vi "ReadType_Bar_AF.vi"(6 "error in":errorcluster, 11 "File Bar":string="C:\\Users\\Hung\\Desktop\\RawData\\New Raw") -> (0 "Linear Velocity (m/s)":dbl, 1 "Gain Max":dbl, 2 "Gain Min":dbl, 3 "Type":i16, 4 "error out":errorcluster, 5 "Linear Move Distance (m)":dbl)   [LabVIEW 2020]
panel:
  out "x/y":dbl
  out "D_Magnetic (mm)":dbl
  out "Simulated Distance":dbl
  out "Duration":dbl
  out "Waveform Graph":dbl[](graph)
  out "V_ship (m/s)":dbl
  out "Voltage Response":dbl
  out "Simulated Distance":i16
  out "D_Magnetic(mm)":i16
  out "Duration":u16
  out "Max ABS Magnetic Value":dbl
  in  "Gain":dbl=1.0 min=-20.0 max=20.0
  out "Data_Double":dbl[](array[numeric])
  out "Number Sample":u32
  out "Size Data":i32
  out "data":i16[](array[numeric])
  in  "file path (use dialog) 2":path=path "C:/Users/Hung/Downloads/filewritefromGUI.bar"
  # "Type 2 is Move Motion\nType 1 is Change Kepco"
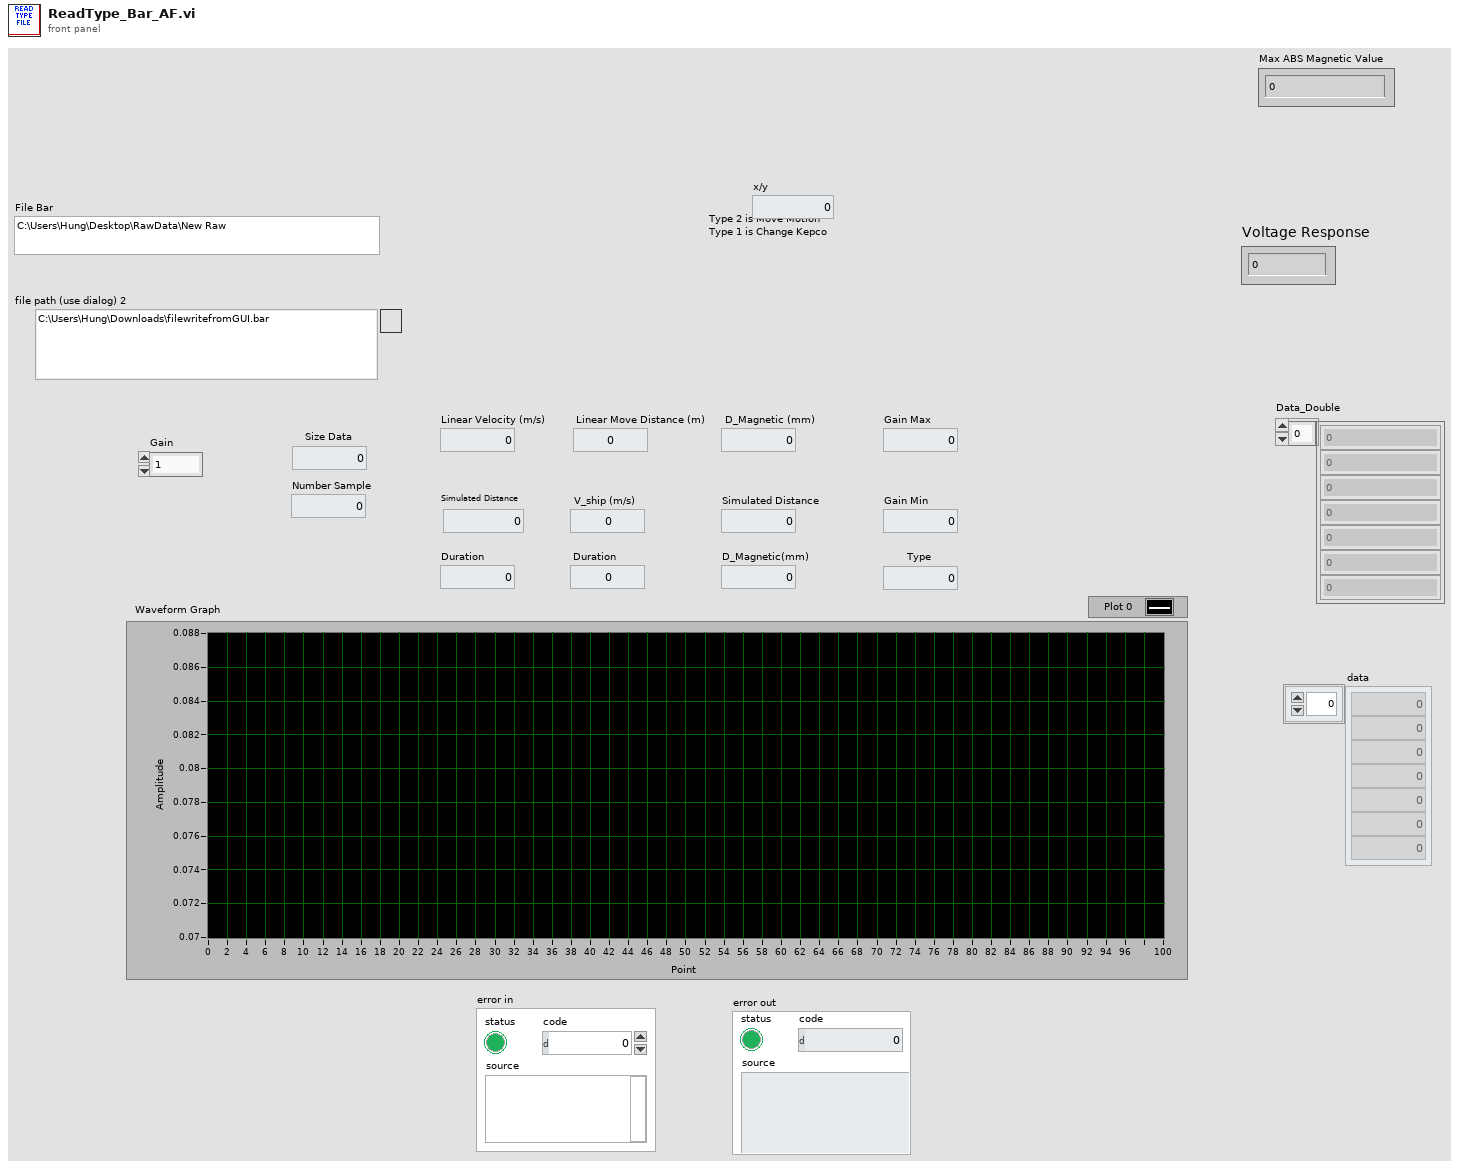
[diagram p1: front panel]
types:
  T1 = enum16{"big-endian, network order", "native, host order", "little-endian"}
  T2 = enum16{"open", "replace", "create", "open or create", "replace or create", "replace or create with confirmation"}
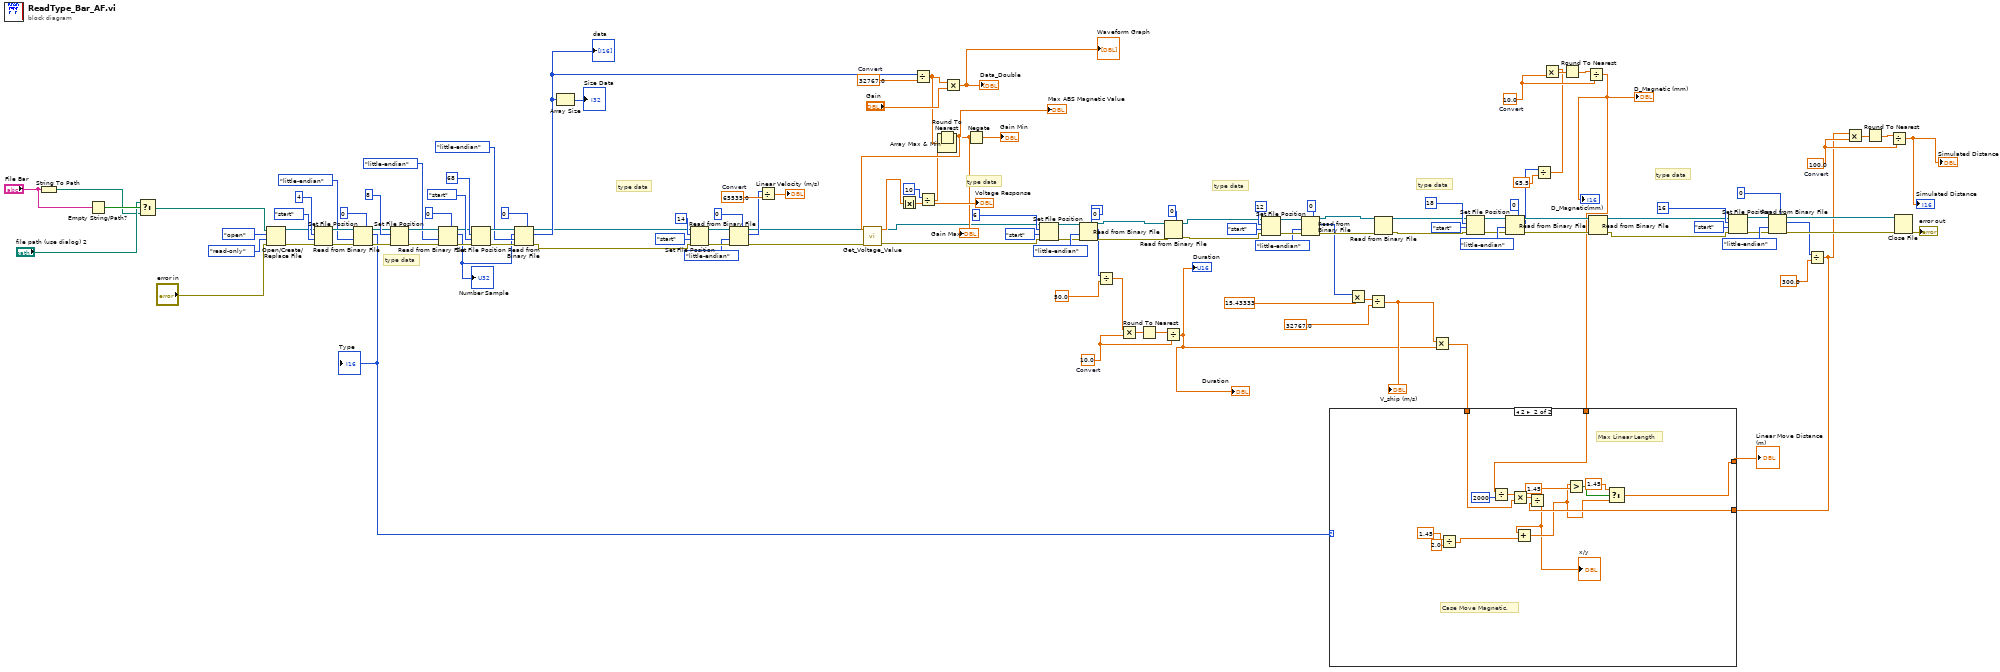
[diagram p0: block diagram]
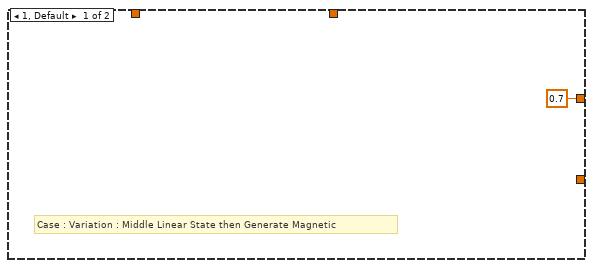
[diagram p2: hidden frame]
diagram:
  w10 = 10.0  # Convert
  w16 = 10.0  # Convert
  w17 = 100.0  # Convert
  w85 = 65535.0  # Convert
  w104 = 32767.0  # Convert
  # "type data"
  # "type data"
  # "type data"
  # "type data"
  # "type data"
  # "type data"
  n1 = String To Path(string="File Bar") -> (path=w26:path)
  n2 = Empty String/Path?(string/path="File Bar") -> (empty?=w28:bool)
  n3 = Select(t="file path (use dialog) 2", s=w28, f=w26) -> (s? t:f=w30:path)
  n4 = Open/Create/Replace File(file path (use dialog)=w30, error in="error in", operation (0:open)=T2."open", access (0:read/write)=enum16{"read/write", "read-only", "write-only"}."read-only") -> (refnum out=w62:refnum<file>, error out=w123:errorcluster)  [unwired: 2 in, 1 out]
  n5 = Set File Position(offset (in bytes) (0)=i64 4, refnum=w62, from (0:start)=enum16{"start", "end", "current"}."start", error in=w123) -> (refnum out=w124:refnum<file>, error out=w122:errorcluster)
  n6 = Read from Binary File(5:i16 0, 8:w122, 9:T1."little-endian" ("byte order (0:big-endian, network order)"), 11:w124) -> (0:w110:errorcluster, 2:w6:i16, 3:w101:refnum<file>)  [unwired: 2 in, 1 out]
  "Type" <- w6
  n7 = Set File Position(offset (in bytes) (0)=i64 8, refnum=w101, error in=w110) -> (refnum out=w112:refnum<file>, error out=w109:errorcluster)  [unwired: 1 in]
  n8 = Read from Binary File(5:u32 0, 8:w109, 9:T1."little-endian" ("byte order (0:big-endian, network order)"), 11:w112) -> (0:w108:errorcluster, 2:w37:u32, 3:w111:refnum<file>)  [unwired: 2 in, 1 out]
  "Number Sample" <- w37
  n9 = Set File Position(offset (in bytes) (0)=i16 68, refnum=w111, from (0:start)=enum16{"start", "end", "current"}."start", error in=w108) -> (refnum out=w117:refnum<file>, error out=w114:errorcluster)
  n10 = Read from Binary File(5:i16 0, 8:w114, 9:T1."little-endian" ("byte order (0:big-endian, network order)"), 10:w37, 11:w117) -> (0:w39:errorcluster, 2:w102:i16[], 3:w38:refnum<file>)  [unwired: 1 in, 1 out]
  "data" <- w102
  n11 = Array Size(array=w102) -> (size(s)=→"Size Data":i32)
  n12 = Set File Position(offset (in bytes) (0)=i64 14, refnum=w38, from (0:start)=enum16{"start", "end", "current"}."start", error in=w39) -> (refnum out=w91:refnum<file>, error out=w88:errorcluster)
  n13 = Read from Binary File(5:u16 0, 8:w88, 9:T1."little-endian" ("byte order (0:big-endian, network order)"), 11:w91) -> (0:w82:errorcluster, 2:w84:u16, 3:w40:refnum<file>)  [unwired: 2 in, 1 out]
  n14 = Divide(x=w84, y=w85) -> (x/y=→"Linear Velocity (m/s)":dbl)
  n15 = Divide(x=w102, y=w104) -> (x/y=w100:dbl[])
  n16 = Array Max & Min(array=w100) -> (max value=w98:dbl)  [unwired: 3 out]
  "Max ABS Magnetic Value" <- w98
  n17 = call "Get_Voltage_Value.vi"("error in"=w82, "Magnetic Field (T)"=w98) -> ("error out"=w41:errorcluster, "Voltage Response"=w97:dbl)  [unwired: 8 in]
  "Voltage Response" <- w97
  n18 = Absolute Value(x=w97) -> (abs(x)=w95:dbl)
  n19 = Divide(x=10, y=w95) -> (x/y=w94:dbl)
  n20 = Round To Nearest(number=w94) -> (nearest integer value=w93:dbl)
  "Gain Max" <- w93
  n21 = Multiply(x=w100, y="Gain") -> (x*y=→"Data_Double" →"Waveform Graph":dbl[])
  n22 = Negate(x=w93) -> (-x=→"Gain Min":dbl)
  n23 = Set File Position(offset (in bytes) (0)=i64 6, refnum=w40, from (0:start)=enum16{"start", "end", "current"}."start", error in=w41) -> (refnum out=w75:refnum<file>, error out=w78:errorcluster)
  n24 = Read from Binary File(5:u16 0, 8:w78, 9:T1."little-endian" ("byte order (0:big-endian, network order)"), 11:w75) -> (0:w60:errorcluster, 2:w24:u16, 3:w1:refnum<file>)  [unwired: 2 in, 1 out]
  n25 = Divide(x=w24, y=50.0) -> (x/y=w9:dbl)
  n26 = Multiply(x=w9, y=w10) -> (x*y=w12:dbl)
  n27 = Round To Nearest(number=w12) -> (nearest integer value=w11:dbl)
  n28 = Read from Binary File(5:i16 0, 8:w60, 11:w1) -> (0:w58:errorcluster, 3:w59:refnum<file>)  [unwired: 3 in, 2 out]
  n29 = Divide(x=w11, y=w10) -> (x/y=w8:dbl)
  "Duration" <- w8
  "Duration" <- w8
  n30 = Set File Position(offset (in bytes) (0)=i64 12, refnum=w59, from (0:start)=enum16{"start", "end", "current"}."start", error in=w58) -> (refnum out=w74:refnum<file>, error out=w71:errorcluster)
  n31 = Read from Binary File(5:i16 0, 8:w71, 9:T1."little-endian" ("byte order (0:big-endian, network order)"), 11:w74) -> (0:w56:errorcluster, 2:w35:i16, 3:w57:refnum<file>)  [unwired: 2 in, 1 out]
  n32 = Multiply(x=w35, y=15.43333) -> (x*y=w34:dbl)
  n33 = Divide(x=w34, y=32767.0) -> (x/y=w32:dbl)
  "V_ship (m/s)" <- w32
  n34 = Read from Binary File(8:w56, 11:w57) -> (0:w54:errorcluster, 3:w55:refnum<file>)  [unwired: 4 in, 2 out]
  n35 = Multiply(x=w32, y=w8) -> (x*y=w3:dbl)
  n36 = Set File Position(offset (in bytes) (0)=i64 18, refnum=w55, from (0:start)=enum16{"start", "end", "current"}."start", error in=w54) -> (refnum out=w63:refnum<file>, error out=w66:errorcluster)
  n37 = Read from Binary File(5:i16 0, 8:w66, 9:T1."little-endian" ("byte order (0:big-endian, network order)"), 11:w63) -> (0:w52:errorcluster, 2:w20:i16, 3:w53:refnum<file>)  [unwired: 2 in, 1 out]
  n38 = Divide(x=w20, y=65.5) -> (x/y=w13:dbl)
  n39 = Multiply(x=w13, y=w16) -> (x*y=w14:dbl)
  n40 = Round To Nearest(number=w14) -> (nearest integer value=w15:dbl)
  n41 = Divide(x=w15, y=w16) -> (x/y=w5:dbl)
  "D_Magnetic(mm)" <- w5
  "D_Magnetic (mm)" <- w5
  n42 = Read from Binary File(8:w52, 11:w53) -> (0:w45:errorcluster, 3:w44:refnum<file>)  [unwired: 4 in, 2 out]
  n43 = Set File Position(offset (in bytes) (0)=i64 16, refnum=w44, from (0:start)=enum16{"start", "end", "current"}."start", error in=w45) -> (refnum out=w46:refnum<file>, error out=w49:errorcluster)
  n44 = Read from Binary File(5:i16 0, 8:w49, 9:T1."little-endian" ("byte order (0:big-endian, network order)"), 11:w46) -> (0:w42:errorcluster, 2:w23:i16, 3:w43:refnum<file>)  [unwired: 2 in, 1 out]
  n45 = Divide(x=w23, y=300.0) -> (x/y=w4:dbl)
  n46 = case shown="2" w6 {
    tunnel: w5 -> [_ w138]
    tunnel: w4 -> [_ w137]
    tunnel: w3 -> [_ w136]
    tunnel: [0.7 ("t") w135] -> w2
    frame 1, Default {
      # "Case : Variation : Middle Linear State then Generate Magnetic"
    }
    frame 2 {
      # "Case Move Magnetic."
      # "Max Linear Length"
      n47 = Divide(x=1.45 ("y"), y=2.0) -> (x/y=w132:dbl)
      n48 = Divide(x=w138, y=i16 2000) -> (x/y=w142:dbl)
      n49 = Multiply(x=w142, y=w136) -> (x*y=w143:dbl)
      n50 = Divide(x=w143, y=w137) -> (x/y=w130:dbl)
      "x/y" <- w130
      n51 = Add(x=w130, y=w132) -> (x+y=w131:dbl)
      n52 = Greater?(x=w131, y=1.45) -> (0:w144:bool)
      n53 = Select(t=1.45, s=w144, f=w131) -> (s? t:f=w135:dbl)
    }
  }
  "Linear Move Distance (m)" <- w2
  n54 = Multiply(x=w4, y=w17) -> (x*y=w19:dbl)
  n55 = Round To Nearest(number=w19) -> (nearest integer value=w18:dbl)
  n56 = Divide(x=w18, y=w17) -> (x/y=→"Simulated Distance" →"Simulated Distance":dbl)
  n57 = Close File(refnum=w43, error in=w42) -> (error out=→"error out":errorcluster)  [unwired: 1 out]
